vi "tdms_bun.vi"() -> ()   [LabVIEW 2020]
panel:
  in  "Multimeter":refnum<visa-resource-name>="GPIB0::7::INSTR"
  in  "Sourcemeter":refnum<visa-resource-name>="GPIB0::5::INSTR"
  out "Vdd":dbl[](array[numeric])
  out "I(OUT)":dbl[](array[numeric])
  out "Idd":sgl[](array[numeric])
  in  "Compliance  Level (0.1)":dbl=0.1 step=0.001
  in  "Pas":dbl
  in  "Max":dbl
  out "error out 2":errorcluster
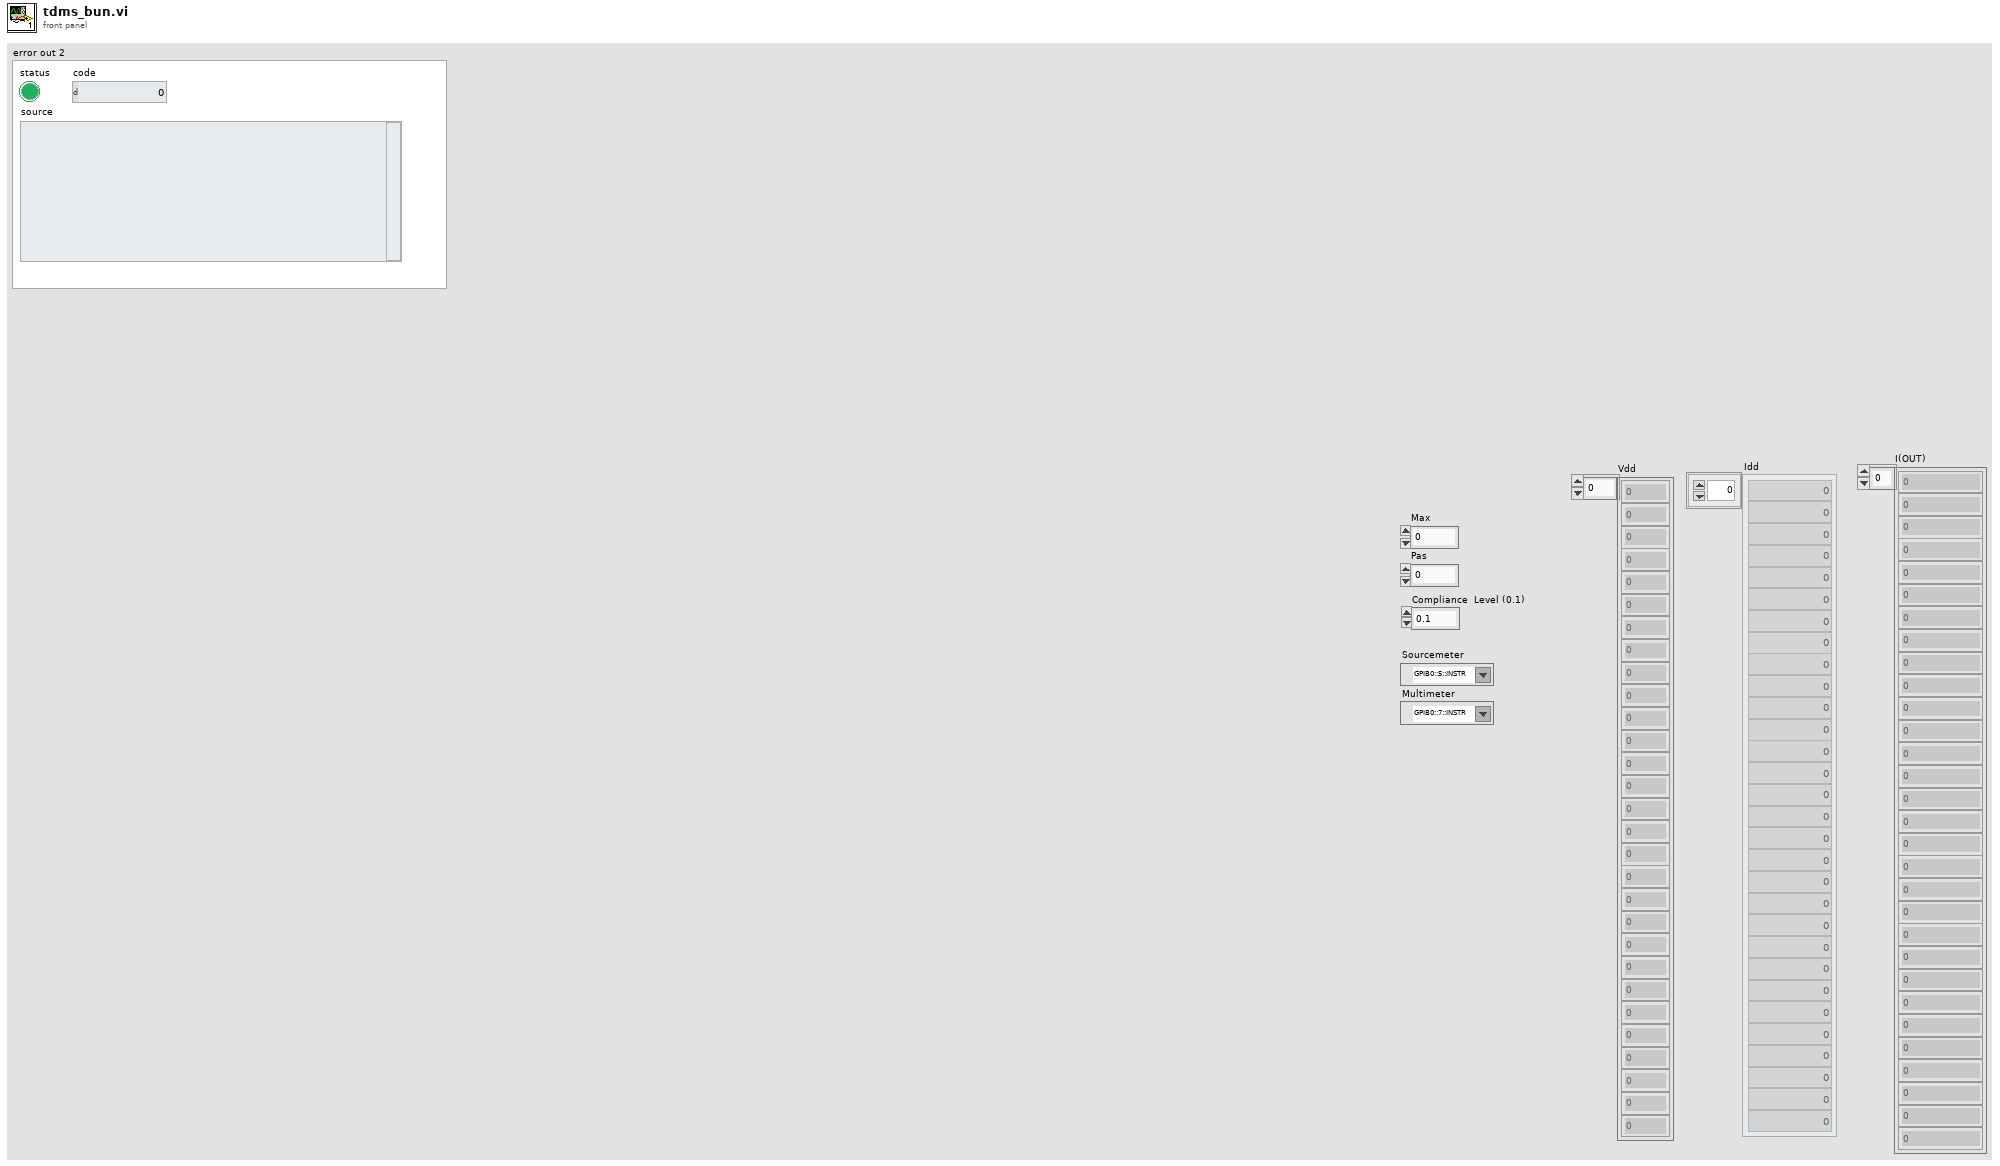
[diagram p1: front panel]
types:
  T1 = enum16{"open", "open or create", "create or replace", "create", "open (read-only)"}
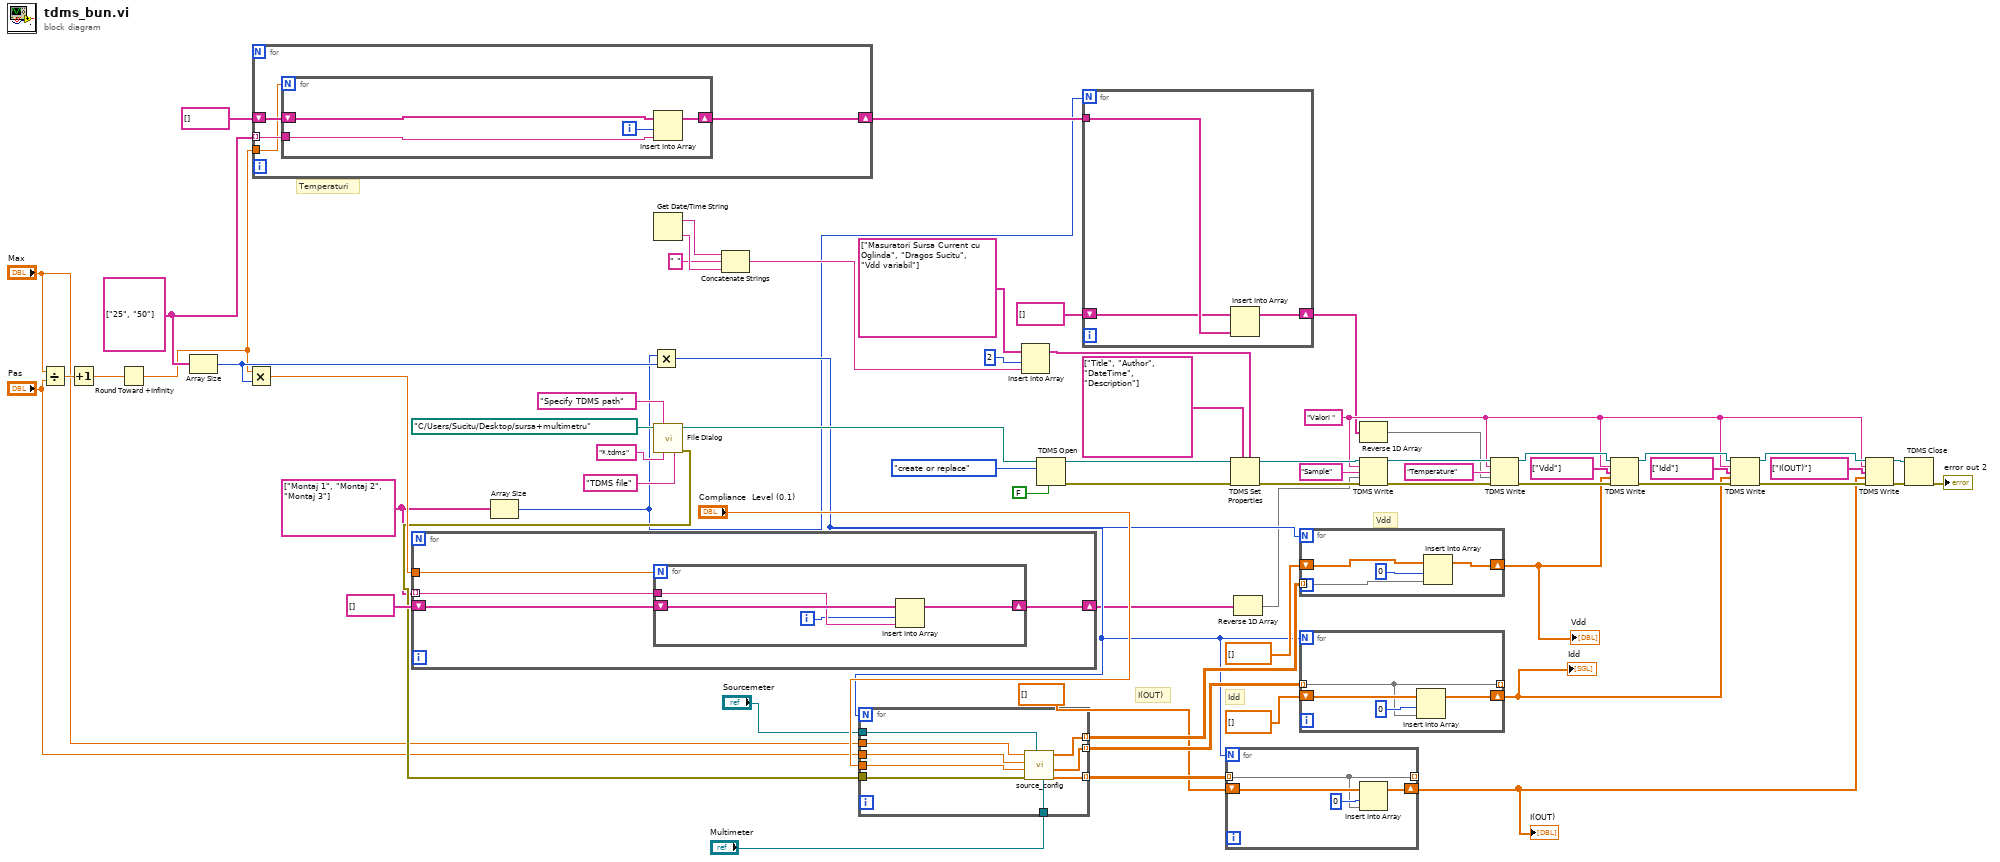
[diagram p0: block diagram]
diagram:
  w13 = string[] ["Montaj 1", "Montaj 2", "Montaj 3"] ("array")
  w30 = string[] ["25", "50"] ("array")
  w40 = "Valori " ("group name in (Untitled)")
  # "I(OUT)"
  # "Idd"
  # "Vdd"
  # "Temperaturi"
  n1 = Divide(x="Max", y="Pas") -> (x/y=w29:dbl)
  n2 = Increment(x=w29) -> (x+1=w28:dbl)
  n3 = Round Toward +Infinity(x=w28) -> (ceil(x): smallest int >= x=w14:dbl)
  n4 = Array Size(array=w30) -> (size(s)=w17:i32)
  n5 = Multiply(x=w14, y=w17) -> (x*y=w26:dbl)
  n6 = for {
    tunnel: w30 -> [w70] mode=indexing
    shift-right: [w71] -> w33
    shift-left: string[] [] -> [w72]
    tunnel: w14 -> [w69]
    n7 = for {
      N: w69 -> [_]
      shift-right: [w76] -> w71
      shift-left: w72 -> [w75]
      tunnel: w70 -> [w74]
      i -> [w73]
      n8 = Insert Into Array(array=w75, index=w73, new element=w74) -> (w76:string[])
    }
  }
  n9 = for {
    tunnel: w13 -> [w78] mode=indexing
    shift-right: [w79] -> w10
    shift-left: string[] [] -> [w80]
    tunnel: w26 -> [w77]
    n10 = for {
      N: w77 -> [_]
      shift-right: [w84] -> w79
      shift-left: w80 -> [w83]
      tunnel: w78 -> [w82]
      i -> [w81]
      n11 = Insert Into Array(array=w83, index=w81, new element=w82) -> (w84:string[])
    }
  }
  n12 = Array Size(array=w13) -> (size(s)=w11:i32)
  n13 = Multiply(x=w11, y=w17) -> (x*y=w12:i32)
  n14 = Get Date/Time String() -> (date string=w59:string, time string=w57:string)  [unwired: 3 in]
  n15 = call "File Dialog"("start path"=path "C:/Users/Sucitu/Desktop/sursa+multimetru", "prompt"="Specify TDMS path", "pattern (all files)"="*.tdms", "pattern label"="TDMS file") -> ("selected path"=w51:path, "error out"=w21:errorcluster)  [unwired: 8 in, 2 out]
  n16 = Concatenate Strings(w59, " " ("string"), w57) -> (w58:string)
  n17 = for {
    N: w12 -> [_]
    tunnel: [w93] -> w25 mode=indexing
    tunnel: [w92] -> w23 mode=indexing
    tunnel: [w91] -> w22 mode=indexing
    tunnel: w21 -> [w90]
    tunnel: "Max" -> [w89]
    tunnel: "Pas" -> [w88]
    tunnel: "Compliance  Level (0.1)" -> [w87]
    tunnel: "Sourcemeter" -> [w86]
    tunnel: "Multimeter" -> [w85]
    n18 = call "source_config.vi"("Multimeter"=w85, "Sourcemeter"=w86, "error in (no error)"=w90, "Compliance  Level (0.1)"=w87, "Pas"=w88, "Max"=w89) -> ("I(OUT)"=w91:dbl[], "Idd"=w92:sgl[], "Vdd"=w93:dbl[])  [unwired: 2 in, 1 out]
  }
  n19 = Insert Into Array(array=string[] ["Masuratori Sursa Current cu Oglinda", "Dragos Sucitu", "Vdd variabil"] ("property names"), index=2, new element=w58) -> (w61:string[])
  n20 = TDMS Open(6:FALSE ("disable buffering? (T)"), 10:T1."create or replace" ("operation (0:open)"), 11:w51) -> (0:w64:errorcluster, 3:w65:refnum<k34>)  [unwired: 4 in]
  n21 = for {
    N: w11 -> [_]
    tunnel: w33 -> [w96]
    shift-right: [w94] -> w31
    shift-left: string[] [] ("array") -> [w95]
    n22 = Insert Into Array(array=w95, new element=w96) -> (w94:string[])  [unwired: 1 in]
  }
  n23 = for {
    N: w12 -> [_]
    shift-right: [w100] -> w5
    shift-left: dbl[] [] -> [w98]
    tunnel: [w97] -> _ mode=indexing
    tunnel: w22 -> [w97] mode=indexing
    n24 = Insert Into Array(array=w98, index=0, new element=w97) -> (w100:dbl[])
  }
  "I(OUT)" <- w5
  n25 = TDMS Set Properties(5:w61, 7:string[] ["Title", "Author", "DateTime", "Description"] ("property names"), 8:w64, 11:w65) -> (0:w49:errorcluster, 3:w50:refnum<k34>)  [unwired: 2 in, 2 out]
  n26 = Reverse 1D Array(array=w10) -> (reversed array=w9:string[])
  n27 = for {
    N: w12 -> [_]
    shift-right: [w104] -> w4
    shift-left: dbl[] [] -> [w101]
    tunnel: w25 -> [w102] mode=indexing
    n28 = Insert Into Array(array=w101, index=0, new element=w102) -> (w104:dbl[])
  }
  "Vdd" <- w4
  n29 = for {
    N: w12 -> [_]
    shift-right: [w108] -> w3
    shift-left: sgl[] [] -> [w106]
    tunnel: [w105] -> _ mode=indexing
    tunnel: w23 -> [w105] mode=indexing
    n30 = Insert Into Array(array=w106, index=0, new element=w105) -> (w108:sgl[])
  }
  "Idd" <- w3
  n31 = Reverse 1D Array(array=w31) -> (reversed array=w15:string[])
  n32 = TDMS Write(0:w50, 5:w40, 7:"Sample" ("channel name(s) in (Untitled)"), 9:w9, 11:w49) -> (4:w48:refnum<k34>, 15:w47:errorcluster)  [unwired: 1 in, 2 out]
  n33 = TDMS Write(0:w48, 5:w40, 7:"Temperature" ("channel name(s) in (Untitled)"), 9:w15, 11:w47) -> (4:w46:refnum<k34>, 15:w45:errorcluster)  [unwired: 1 in, 2 out]
  n34 = TDMS Write(0:w46, 5:w40, 7:string[] ["Vdd"] ("channel name(s) in (Untitled)"), 9:w4, 11:w45) -> (4:w44:refnum<k34>, 15:w43:errorcluster)  [unwired: 1 in, 2 out]
  n35 = TDMS Write(0:w44, 5:w40, 7:string[] ["Idd"] ("channel name(s) in (Untitled)"), 9:w3, 11:w43) -> (4:w42:refnum<k34>, 15:w41:errorcluster)  [unwired: 1 in, 2 out]
  n36 = TDMS Write(0:w42, 5:w40, 7:string[] ["I(OUT)"] ("channel name(s) in (Untitled)"), 9:w5, 11:w41) -> (4:w35:refnum<k34>, 15:w36:errorcluster)  [unwired: 1 in, 2 out]
  n37 = TDMS Close(8:w36, 11:w35) -> (0:→"error out 2":errorcluster)  [unwired: 1 out]
